vi "APC_9056_TEMPLATEControl.vi"(1 "PC_ControlSettings":T1={"Spark advance [CADBTDC]"=0.0, "Pref"=0.0, "O2ref"=0.0, "DI advance [CADBTDC]"=0.0, "DI duration [ms] "=0.0, "CO2ref"=0.0, "PFI advance [CADBTDC]"=0.0, "PFI duration [ms]"=0.0, "IMEP ref"=0.0, "Speed ref"=1800.0, "IGN enable"=TRUE, "DI enable"=TRUE, "CL PFI\n lambda"=FALSE, "CL PFI\nIMEP"=FALSE, "Activate\ncylinder"=[FALSE, FALSE, FALSE, FALSE, FALSE, FALSE], "Force idling"=FALSE, "Force motoring"=FALSE, "ETP resync"=FALSE, "Requested mode"=0, "Clear Sync Errors"=FALSE, "toggle TDC"=FALSE, "l ref"=0.0, "PID control references"={"NG"=FALSE, "Ar"=FALSE, "O2"=FALSE, "Intake vent"=FALSE, "Cross vent"=FALSE, "Exhaust vent"=FALSE, "NG control mode"=0, "NG-FC-001-REF"=0.0, "WF-OA-002-REF"=0.0, "IMEP-REF"=0.0, "Nm-REF"=0.0, "Ar control mode"=0, "N-PC-002-REF"=0.0, "WF-PT-004-REF"=0.0, "O2 control mode"=0, "O2-FC-001-REF"=0.0, "WF-OA-001-REF"=0.0, "Tcoolant control  mode"=0, "EC-FC-001-REF"=0.0, "EC-TT-001-REF"=0.0, "Texh control mode"=0, "SW-FC-004-REF"=0.0, "SW-FT-002-REF"=0.0, "WF-TT-004-REF"=0.0, "Toil control mode"=0, "SW-FC-009-REF"=0.0, "SW-FT-004-REF"=0.0, "EO-TT-001-REF"=0.0, "AIC201_CO2_ConcTarget"=0.0, "O2_FF_NG"=FALSE, "Dyno control mode"=0, "Membrane control mode"=0, "AR-FT-001-REF"=0.0, "MTR modbus floats"=[0.0, 0.0, 0.0, 0.0, 0.0, 0.0, 0.0, 0.0, 0.0, 0.0, 0.0, 0.0, 0.0, 0.0, 0.0, 0.0, 0.0, 0.0, 0.0], "MTR modbus u16"=[0, 0, 0, 0, 0, 0, 0], "MTR HB"=FALSE, "PC_HB"=FALSE, "EMERGENCY STOP"=FALSE}, "CA50setpoint [CADATDC]"=0.0, "CA50 control"=TRUE, "Knock control"=FALSE, "CLEAR EMERGENCY STOP"=FALSE, "EMERGENCY STOP"=FALSE}, 2 "input cluster":T3) -> (0 "SW-FC-004-REF":dbl format="%.2f")   [LabVIEW 2020]
uses:
  controls/APC_PIDCluster.ctl
  controls/APC_ControlSettings.ctl
  controls/APC_PIDcontrolSettings.ctl
  controls/APC_cascadePIDsettings.ctl
  <vilib>/addons/control/pid/pid.llb/PID Advanced (DBL).vi
  <vilib>/Utility/xml.llb/Write to XML File(string).vi
  <vilib>/Utility/xml.llb/Read From XML File(string).vi
  <vilib>/addons/control/pid/NI_PID_pid.lvlib
panel:
  in  "save":bool
  in  "load":bool
  out "Texh control mode":u8
  out "EC-FC-001":dbl
  in  "LL FF control":dbl format="%.2f"
  in  "reinitialize LL? (F)":bool
  out "EC-TT-001":dbl
  in  "EC-FC-001-REF (manual)":dbl
  in  "EC-TT-001-REF (manual)":dbl
  in  "Texh control mode (manual)":u8
  out "HL on?":bool
  out "HL setpoint":dbl format="%.2f"
  in  "LL PID gains":T4={"proportional gain (Kc)"=1.0, "integral time (Ti, min)"=0.01, "derivative time (Td, min)"=0.0} {"derivative time (Td, min)" format="%.3f"; "integral time (Ti, min)" format="%.3f"; "proportional gain (Kc)" format="%.3f"}
  in  "LL PID setpoint range":cluster{"setpoint high":dbl, "setpoint low":dbl}={"setpoint high"=100.0, "setpoint low"=0.0} {"setpoint high" format="%.2f"; "setpoint low" format="%.2f"}
  in  "LL PID output range":cluster{"output high":dbl, "output low":dbl}={"output high"=100.0, "output low"=-100.0} {"output low" format="%.2f"; "output high" format="%.2f"}
  in  "Override PC PID references":bool
  in  "HL learn?":bool=TRUE
  in  "HL FF control":dbl format="%.2f"
  in  "HL PID gains":T4={"proportional gain (Kc)"=1.0, "integral time (Ti, min)"=0.01, "derivative time (Td, min)"=0.0} {"derivative time (Td, min)" format="%.3f"; "integral time (Ti, min)" format="%.3f"; "proportional gain (Kc)" format="%.3f"}
  in  "HL PID setpoint range":cluster{"setpoint high":dbl, "setpoint low":dbl}={"setpoint high"=100.0, "setpoint low"=0.0} {"setpoint high" format="%.2f"; "setpoint low" format="%.2f"}
  in  "HL PID output range":cluster{"output high":dbl, "output low":dbl}={"output high"=100.0, "output low"=-100.0} {"output low" format="%.2f"; "output high" format="%.2f"}
  in  "Safe mode control":dbl format="%.2f"
  in  "LL learn?":bool=TRUE
  in  "reinitialize HL? (F)":bool
  out "LL on?":bool
  out "LL setpoint":dbl format="%.2f"
  # "Texh control"
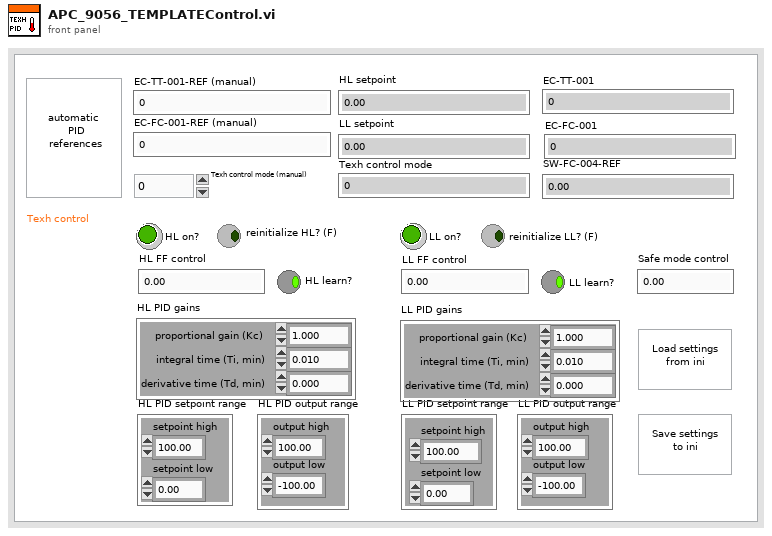
[diagram p1: front panel]
types:
  T1 = typedef "APC_ControlSettings.ctl" = cluster{"Spark advance [CADBTDC]":dbl, "Pref":dbl, "O2ref":dbl, "DI advance [CADBTDC]":dbl, "DI duration [ms] ":dbl, "CO2ref":dbl, "PFI advance [CADBTDC]":dbl, "PFI duration [ms]":dbl, "IMEP ref":dbl, "Speed ref":dbl, "IGN enable":bool, "DI enable":bool, "CL PFI\n lambda":bool, "CL PFI\nIMEP":bool, "Activate\ncylinder":bool[], "Force idling":bool, "Force motoring":bool, "ETP resync":bool, "Requested mode":i8, "Clear Sync Errors":bool, "toggle TDC":bool, "l ref":dbl, "PID control references":T2, "CA50setpoint [CADATDC]":dbl, "CA50 control":bool, "Knock control":bool, "CLEAR EMERGENCY STOP":bool, "EMERGENCY STOP":bool}
  T2 = typedef "APC_PIDcontrolSettings.ctl" = cluster{"NG":bool, "Ar":bool, "O2":bool, "Intake vent":bool, "Cross vent":bool, "Exhaust vent":bool, "NG control mode":u8, "NG-FC-001-REF":dbl, "WF-OA-002-REF":dbl, "IMEP-REF":dbl, "Nm-REF":dbl, "Ar control mode":u8, "N-PC-002-REF":dbl, "WF-PT-004-REF":dbl, "O2 control mode":u8, "O2-FC-001-REF":dbl, "WF-OA-001-REF":dbl, "Tcoolant control  mode":u8, "EC-FC-001-REF":dbl, "EC-TT-001-REF":dbl, "Texh control mode":u8, "SW-FC-004-REF":dbl, "SW-FT-002-REF":dbl, "WF-TT-004-REF":dbl, "Toil control mode":u8, "SW-FC-009-REF":dbl, "SW-FT-004-REF":dbl, "EO-TT-001-REF":dbl, "AIC201_CO2_ConcTarget":dbl, "O2_FF_NG":bool, "Dyno control mode":u8, "Membrane control mode":u8, "AR-FT-001-REF":dbl, "MTR modbus floats":sgl[], "MTR modbus u16":u16[], "MTR HB":bool, "PC_HB":bool, "EMERGENCY STOP":bool}
  T3 = typedef "APC_PIDCluster.ctl" = cluster{"AR-FT-001":dbl, "O2-FC-001":dbl, "SW-FT-004":dbl, "SW-FT-002":dbl, "WF-OA-002":dbl, "WF-PT-004":dbl, "WF-OA-001":dbl, "EC-TT-001":dbl, "WF-TT-004":dbl, "EC-FC-001":dbl, "NG-FC-001":dbl, "EO-TT-001":dbl, "SW-FC-008":dbl, "SW-FC-004":dbl, "IMEPn6":dbl, "TORQUE":dbl, "CylPresWarnings":dbl, "CylPresErrors":dbl, "NG-FT-001":dbl, "EngineSpeed_rpm":dbl}
  T4 = cluster{"proportional gain (Kc)":dbl, "integral time (Ti, min)":dbl, "derivative time (Td, min)":dbl}
  T5 = typedef "APC_cascadePIDsettings.ctl" = cluster{"HL FF control":dbl, "LL FF control":dbl, "HL PID gains":cluster{"proportional gain (Kc)":dbl, "integral time (Ti, min)":dbl, "derivative time (Td, min)":dbl}, "LL PID gains":cluster{"proportional gain (Kc)":dbl, "integral time (Ti, min)":dbl, "derivative time (Td, min)":dbl}, "HL PID setpoint range":cluster{"setpoint high":dbl, "setpoint low":dbl}, "HL PID output range":cluster{"output high":dbl, "output low":dbl}, "LL PID setpoint range":cluster{"setpoint high":dbl, "setpoint low":dbl}, "LL PID output range":cluster{"output high":dbl, "output low":dbl}, "Safe mode control":dbl}
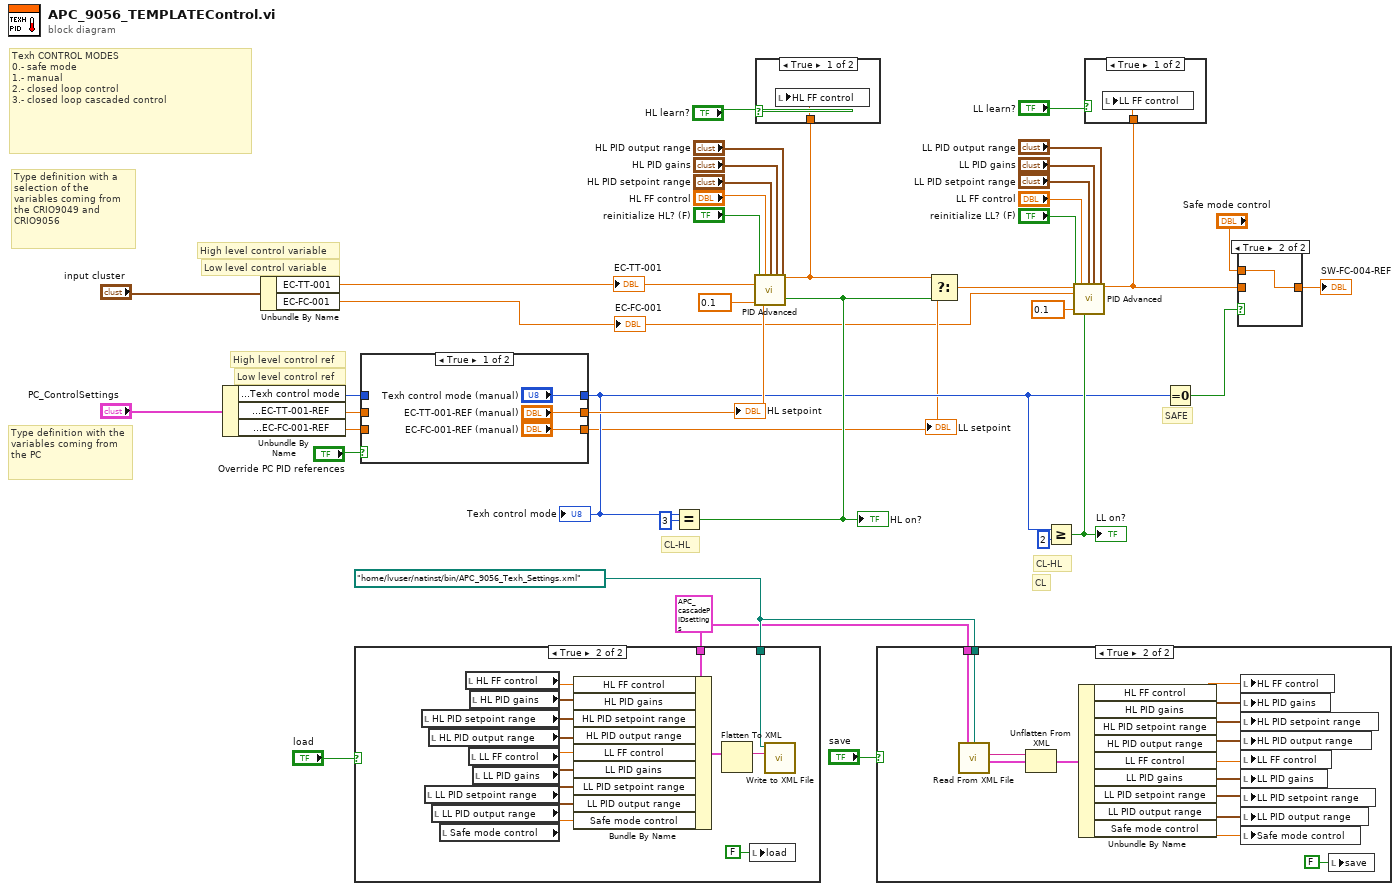
[diagram p0: block diagram]
diagram:
  w4 = path "/home/lvuser/natinst/bin/APC_9056_Texh_Settings.xml" ("XML File Path")
  w3 = T5 {"HL FF control"=0.0, "LL FF control"=0.0, "HL PID gains"={"proportional gain (Kc)"=1.0, "integral time (Ti, min)"=0.01, "derivative time (Td, min)"=0.0}, "LL PID gains"={"proportional gain (Kc)"=1.0, "integral time (Ti, min)"=0.01, "derivative time (Td, min)"=0.0}, "HL PID setpoint range"={"setpoint high"=100.0, "setpoint low"=0.0}, "HL PID output range"={"output high"=0.0, "output low"=0.0}, "LL PID setpoint range"={"setpoint high"=100.0, "setpoint low"=0.0}, "LL PID output range"={"output high"=10.0, "output low"=-10.0}, "Safe mode control"=0.0} ("Cluster")
  # "Type definition with a selection of the variables coming from the CRIO9049 and CRIO9056"
  # "Type definition with the variables coming from the PC"
  # "CL-HL"
  # "Low level control ref"
  # "Low level control variable"
  # "High level control ref"
  # "High level control variable"
  # "SAFE"
  # "CL-HL"
  # "CL"
  # "Texh CONTROL MODES\n0.- safe mode\n1.- manual\n2.- closed loop control \n3.- closed loop cascaded control"
  n1 = Unbundle By Name("PC_ControlSettings") -> ("PID control references.Texh control mode"=w15:u8, "PID control references.EC-TT-001-REF"=w14:dbl, "PID control references.EC-FC-001-REF"=w13:dbl)
  n2 = Unbundle By Name("input cluster") -> ("EC-TT-001"=w12:dbl, "EC-FC-001"=w7:dbl)
  "EC-TT-001" <- w12
  "EC-FC-001" <- w7
  n3 = case shown="True" "load" {
    tunnel: w4 -> [_ w42]
    tunnel: w3 -> [_ w41]
    frame False {
    }
    frame True {
      n4 = local read "HL PID setpoint range"() -> (w51:cluster{"setpoint high":dbl, "setpoint low":dbl})
      n5 = local read "LL PID setpoint range"() -> (w47:cluster{"setpoint high":dbl, "setpoint low":dbl})
      n6 = local read "HL PID output range"() -> (w50:cluster{"output high":dbl, "output low":dbl})
      n7 = local read "LL PID output range"() -> (w46:cluster{"output high":dbl, "output low":dbl})
      n8 = local read "Safe mode control"() -> (w45:dbl)
      n9 = local read "HL FF control"() -> (w53:dbl)
      n10 = local read "LL FF control"() -> (w49:dbl)
      n11 = local read "HL PID gains"() -> (w52:T4)
      n12 = local read "LL PID gains"() -> (w48:T4)
      n13 = Bundle By Name(cluster=w41, "HL FF control"=w53, "HL PID gains"=w52, "HL PID setpoint range"=w51, "HL PID output range"=w50, "LL FF control"=w49, "LL PID gains"=w48, "LL PID setpoint range"=w47, "LL PID output range"=w46, "Safe mode control"=w45) -> (w44:T5)
      n14 = Flatten To XML(6:w44) -> (2:w43:string)
      n15 = local write "load"(FALSE ("load")) -> ()
      n16 = call-poly <vilib>:"Write to XML File.vi"("XML Input"=w43, "XML File Path"=w42) -> ()  [unwired: 7 in, 3 out]
    }
  }
  n17 = case shown="True" "Override PC PID references" {
    tunnel: w15 -> [_ w59]
    tunnel: w14 -> [_ w58]
    tunnel: w13 -> [_ w57]
    tunnel: ["Texh control mode (manual)" w59] -> w10
    tunnel: ["EC-TT-001-REF (manual)" w58] -> w11
    tunnel: ["EC-FC-001-REF (manual)" w57] -> w9
    frame True {
    }
    frame False {
    }
  }
  "LL setpoint" <- w9
  "HL setpoint" <- w11
  "Texh control mode" <- w10
  n18 = Equal?(x=w10, y=u8 3) -> (x = y?=w22:bool)
  "HL on?" <- w22
  n19 = call-poly <vilib>:"PID Advanced.vi"("setpoint"=w11, "output range"="HL PID output range", "auto? (T)"=w22, "manual control"="HL FF control", "process variable"=w12, "setpoint range"="HL PID setpoint range", "PID gains"="HL PID gains", "dt (s)"=0.1, "reinitialize? (F)"="reinitialize HL? (F)") -> ("output"=w27:dbl)  [unwired: 5 in, 1 out]
  n20 = case shown="True" "HL learn?" {
    tunnel: w27 -> [w60 _]
    frame True {
      n21 = local write "HL FF control"(w60) -> ()
    }
    frame False {
    }
  }
  n22 = case shown="True" "save" {
    tunnel: w4 -> [_ w73]
    tunnel: w3 -> [_ w72]
    frame False {
    }
    frame True {
      n23 = call-poly <vilib>:"Read From XML File.vi"("XML File Path"=w73) -> ("XML Elements"=w74:string)  [unwired: 8 in, 2 out]
      n24 = Unflatten From XML(xml string=w74, type=w72) -> (value=w71:T5)  [unwired: 1 in, 1 out]
      n25 = Unbundle By Name(w71) -> ("HL FF control"=w70:dbl, "HL PID gains"=w69:T4, "HL PID setpoint range"=w68:cluster{"setpoint high":dbl, "setpoint low":dbl}, "HL PID output range"=w67:cluster{"output high":dbl, "output low":dbl}, "LL FF control"=w66:dbl, "LL PID gains"=w65:T4, "LL PID setpoint range"=w64:cluster{"setpoint high":dbl, "setpoint low":dbl}, "LL PID output range"=w63:cluster{"output high":dbl, "output low":dbl}, "Safe mode control"=w62:dbl)
      n26 = local write "HL FF control"(w70) -> ()
      n27 = local write "HL PID gains"(w69) -> ()
      n28 = local write "HL PID setpoint range"(w68) -> ()
      n29 = local write "HL PID output range"(w67) -> ()
      n30 = local write "LL FF control"(w66) -> ()
      n31 = local write "LL PID gains"(w65) -> ()
      n32 = local write "LL PID setpoint range"(w64) -> ()
      n33 = local write "LL PID output range"(w63) -> ()
      n34 = local write "Safe mode control"(w62) -> ()
      n35 = local write "save"(FALSE ("save")) -> ()
    }
  }
  n36 = Select(t=w27, s=w22, f=w9) -> (s? t:f=w33:dbl)
  n37 = Greater Or Equal?(x=w10, y=u8 2) -> (x >= y?=w36:bool)
  "LL on?" <- w36
  n38 = call-poly <vilib>:"PID Advanced.vi"("setpoint"=w33, "output range"="LL PID output range", "auto? (T)"=w36, "manual control"="LL FF control", "process variable"=w7, "setpoint range"="LL PID setpoint range", "PID gains"="LL PID gains", "dt (s)"=0.1, "reinitialize? (F)"="reinitialize LL? (F)") -> ("output"=w39:dbl)  [unwired: 5 in, 1 out]
  n39 = case shown="True" "LL learn?" {
    tunnel: w39 -> [w75 _]
    frame True {
      n40 = local write "LL FF control"(w75) -> ()
    }
    frame False {
    }
  }
  n41 = Equal To 0?(x=w10) -> (x = 0?=w38:bool)
  n42 = case shown="True" w38 {
    tunnel: [w76 w77] -> w21
    tunnel: "Safe mode control" -> [_ w77]
    tunnel: w39 -> [w76 _]
    frame False {
    }
    frame True {
    }
  }
  "SW-FC-004-REF" <- w21
